vi "ENUM_Build Array of each Item.vi"(4 "Enum":variant) -> (1 "Enum Array Out":variant[](array[variant]))   [LabVIEW 2015]
doc: "Returns Enum Strings array, String Value and Enum Name from an Enum."
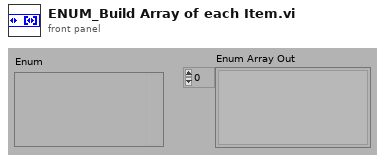
[diagram p1: front panel]
types:
  T1 = typedef "Type Descriptor Header.ctl" = cluster{"length":u16, "private":u8, "type":T2, "# elements":u16}
  T2 = typedef "Type Descriptor Enumeration.ctl" = enum8{"<Null>", "I8", "I16", "I32", "I64", "U8", "U16", "U32", "U64", "SGL", "DBL", "EXT", "CSG", "CDB", "CXT", "0x0F", "0x10", "0x11", "0x12", "0x13", "0x14", "Enum U8", "Enum U16", "Enum U32", "Enum U64", "SGL PQ", "DBL PQ", "EXT PQ", "CSG PQ", "CDB PQ", "CXT PQ", "0x1F", "0x20", "Boolean", "0x22", "0x23", "0x24", "0x25", "0x26", "0x27", "0x28", "0x29", "0x2A", "0x2B", "0x2C", "0x2D", "0x2E", "0x2F", "String", "0x31", "Path", "Pict", "0x34", "0x35", "0x36", "DAQ", "0x38", "0x39", "0x3A", "0x3B", "0x3C", "0x3D", "0x3E", "0x3F", "Array", "0x41", "0x42", "0x43", "0x44", "0x45", "0x46", "0x47", "0x48", "0x49", "0x4A", "0x4B", "0x4C", "0x4D", "0x4E", "0x4F", "Cluster", "0x51", "0x52", "Variant", "Waveform", "0x55", "0x56", "0x57", "0x58", "0x59", "0x5A", "0x5B", "0x5C", "0x5D", "0x5E", "0x5F", "0x60", "0x61", "0x62", "0x63", "0x64", "0x65", "0x66", "0x67", "0x68", "0x69", "0x6A", "0x6B", "0x6C", "0x6D", "0x6E", "0x6F", "Refnum"}
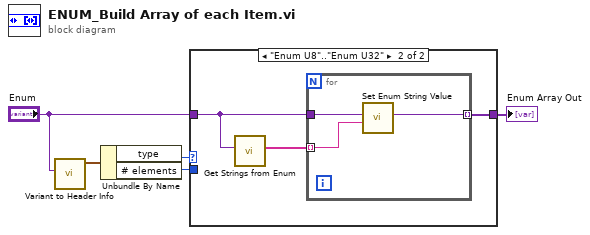
[diagram p0: block diagram]
diagram:
  n1 = call "Variant to Header Info.vi"("Variant"="Enum") -> ("Type Descriptor Header"=w5:T1)  [unwired: 3 in, 2 out]
  n2 = Unbundle By Name(w5) -> ("type"=w4:T2, "# elements"=w3:u16)
  n3 = case shown="\"Enum U8\"..\"Enum U32\"" w4 {
    tunnel: w3 -> [_ _]
    tunnel: "Enum" -> [_ w8]
    tunnel: [_ w6] -> w1
    frame Default {
    }
    frame "Enum U8".."Enum U32" {
      n4 = call "Get Strings from Enum.vi"("Enum"=w8) -> ("Enum Strings"=w7:string[])  [unwired: 7 in, 3 out]
      n5 = for {
        tunnel: w8 -> [w11]
        tunnel: w7 -> [w10] mode=indexing
        tunnel: [w9] -> w6 mode=indexing
        n6 = call "Set Enum String Value.vi"("String Value"=w10, "Default Enum Value"=w11) -> ("Enum"=w9:variant)  [unwired: 8 in, 1 out]
      }
    }
  }
  "Enum Array Out" <- w1
